vi "Initialize Gain.vi"(8 "error in (no error)":errorcluster, 11 "Instrument.Lockin":refnum<class "Instrument.Lockin.lvclass">) -> (0 "error out":errorcluster, 2 "Gain":dbl[](array[numeric]), 3 "Instrument.Lockin out":refnum<class "Instrument.Lockin.lvclass">)   [LabVIEW 2016, in "Instrument.Lockin.lvclass"]
uses:
  Instrument.Lockin.lvclass
  Instrument.Lockin.lvclass/Instrument.Lockin.ctl
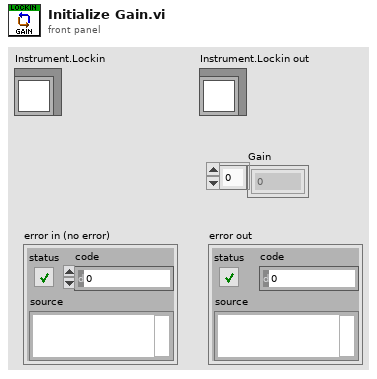
[diagram p1: front panel]
types:
  T1 = typedef "LockinDAQ.lvclass/AO.config-array.ctl" = T2[]
  T2 = typedef "LockinDAQ.lvclass/AO.config-cluster.ctl" = cluster{"AO.channels":tag, "AO.Range":T3, "output terminal configuration":i32, "DAQ Type":T4}
  T3 = typedef "LockinDAQ.lvclass/446xAO-enum.ctl" = enum16{"±0.1 V", "±1.0 V", "±10.0 V"}
  T4 = typedef "LockinDAQ.lvclass/DAQType-enum.ctl" = enum16{"None", "USB 4431", "PXI 446x"}
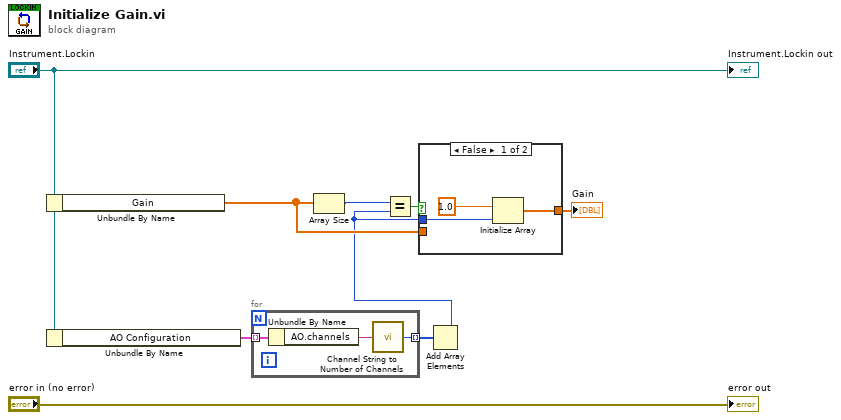
[diagram p0: block diagram]
diagram:
  n1 = Unbundle By Name("Instrument.Lockin") -> ("Gain"=w9:dbl[])
  n2 = Unbundle By Name("Instrument.Lockin") -> ("AO Configuration"=w8:T1)
  n3 = for {
    tunnel: w8 -> [w12] mode=indexing
    tunnel: [w10] -> w4 mode=indexing
    n4 = Unbundle By Name(w12) -> ("AO.channels"=w11:tag)
    n5 = call "Channel String to Number of Channels.vi"("Channels String"=w11) -> ("# channels"=w10:i32)  [unwired: 4 in]
  }
  n6 = Array Size(array=w9) -> (size(s)=w5:i32)
  n7 = Add Array Elements(numeric array=w4) -> (sum=w7:i32)
  n8 = Equal?(x=w5, y=w7) -> (x = y?=w6:bool)
  n9 = case shown="False" w6 {
    tunnel: [w13 w16] -> w1
    tunnel: w9 -> [_ w16]
    tunnel: w7 -> [w14 _]
    frame False {
      n10 = Initialize Array(1.0, w14) -> (w13:dbl[])
    }
    frame True {
    }
  }
  "Gain" <- w1
  "Instrument.Lockin out" <- "Instrument.Lockin"
  "error out" <- "error in (no error)"
